vi "close_data_log.vi"(8 "error in (no error)":errorcluster, 11 "hdf5_photon_record_log in":refnum<class "hdf5_photon_record_log.lvclass">) -> (0 "error out":errorcluster, 3 "hdf5_photon_record_log out":refnum<class "hdf5_photon_record_log.lvclass">)   [LabVIEW 2015, in "hdf5_photon_record_log.lvclass"]
uses:
  hdf5_photon_record_log.lvclass
  hdf5_photon_record_log.lvclass/hdf5_photon_record_log.ctl
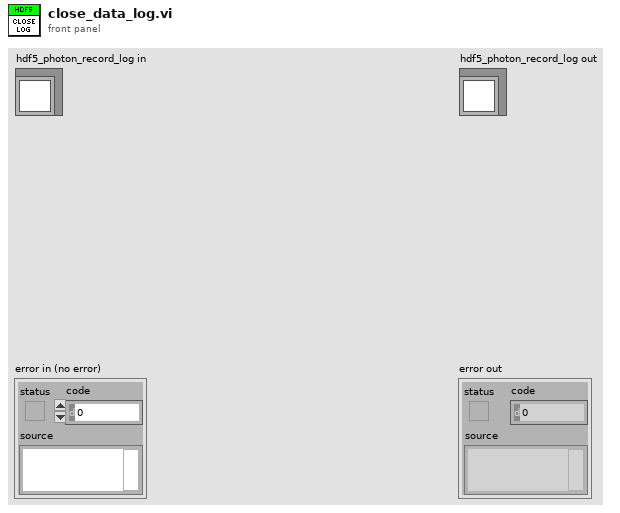
[diagram p1: front panel]
types:
  T1 = typedef "HDF5 Ref.ctl" = refnum<k1>
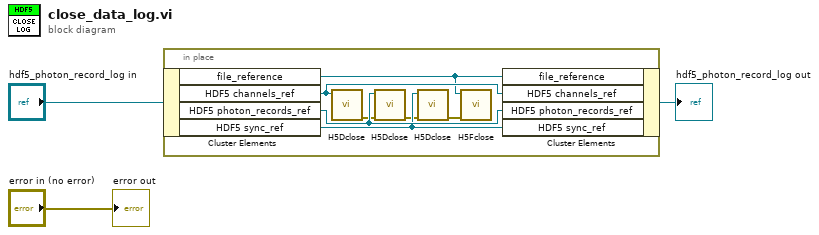
[diagram p0: block diagram]
diagram:
  n1 = in-place {
    n2 = in-place-cluster #1("hdf5_photon_record_log in") -> ("file_reference"=w9:T1, "HDF5 channels_ref"=w10:T1, "HDF5 photon_records_ref"=w8:T1, "HDF5 sync_ref"=w7:T1)
    n3 = call <vilib>:"H5Dclose.vi"("HDF5 Dataset Ref"=w10) -> ("error out"=w6:errorcluster)  [unwired: 8 in]
    n4 = call <vilib>:"H5Dclose.vi"("error in (no error)"=w6, "HDF5 Dataset Ref"=w8) -> ("error out"=w5:errorcluster)  [unwired: 7 in]
    n5 = call <vilib>:"H5Dclose.vi"("error in (no error)"=w5, "HDF5 Dataset Ref"=w7) -> ("error out"=w4:errorcluster)  [unwired: 7 in]
    n6 = call <vilib>:"H5Fclose.vi"("error in (no error)"=w4, "HDF5 Ref"=w9) -> ()  [unwired: 7 in, 1 out]
    n7 = in-place-cluster #1("file_reference"=w9, "HDF5 channels_ref"=w10, "HDF5 photon_records_ref"=w8, "HDF5 sync_ref"=w7) -> (→"hdf5_photon_record_log out":refnum<class "hdf5_photon_record_log.lvclass">)
  }
  "error out" <- "error in (no error)"
